vi "Start Preview.vi"(0 "Cluster In":T3, 1 "Start?":bool, 2 "Info":refnum<vi>, 3 "Stop":refnum<vi>, 4 "Pause":refnum<vi>, 5 "Run":refnum<vi>, 8 "Grab Window Image":refnum<vi>) -> (6 "Cluster Out":T3)   [LabVIEW 2010]
uses:
  System.Windows.Forms
  drivers/DirectShow SDK/v10/DirectShow SDK.llb/DirectShow - Capture Device.ctl
  D:/Projekte/Promotion/Scripts/LabView/drivers/DirectShow SDK/lib/DirectShowLib-2005.dll
  drivers/DirectShow SDK/lib/DirectShowLib-2005.dll
  drivers/DirectShow SDK/v10/DirectShow SDK.llb/DirectShow - Media State.ctl
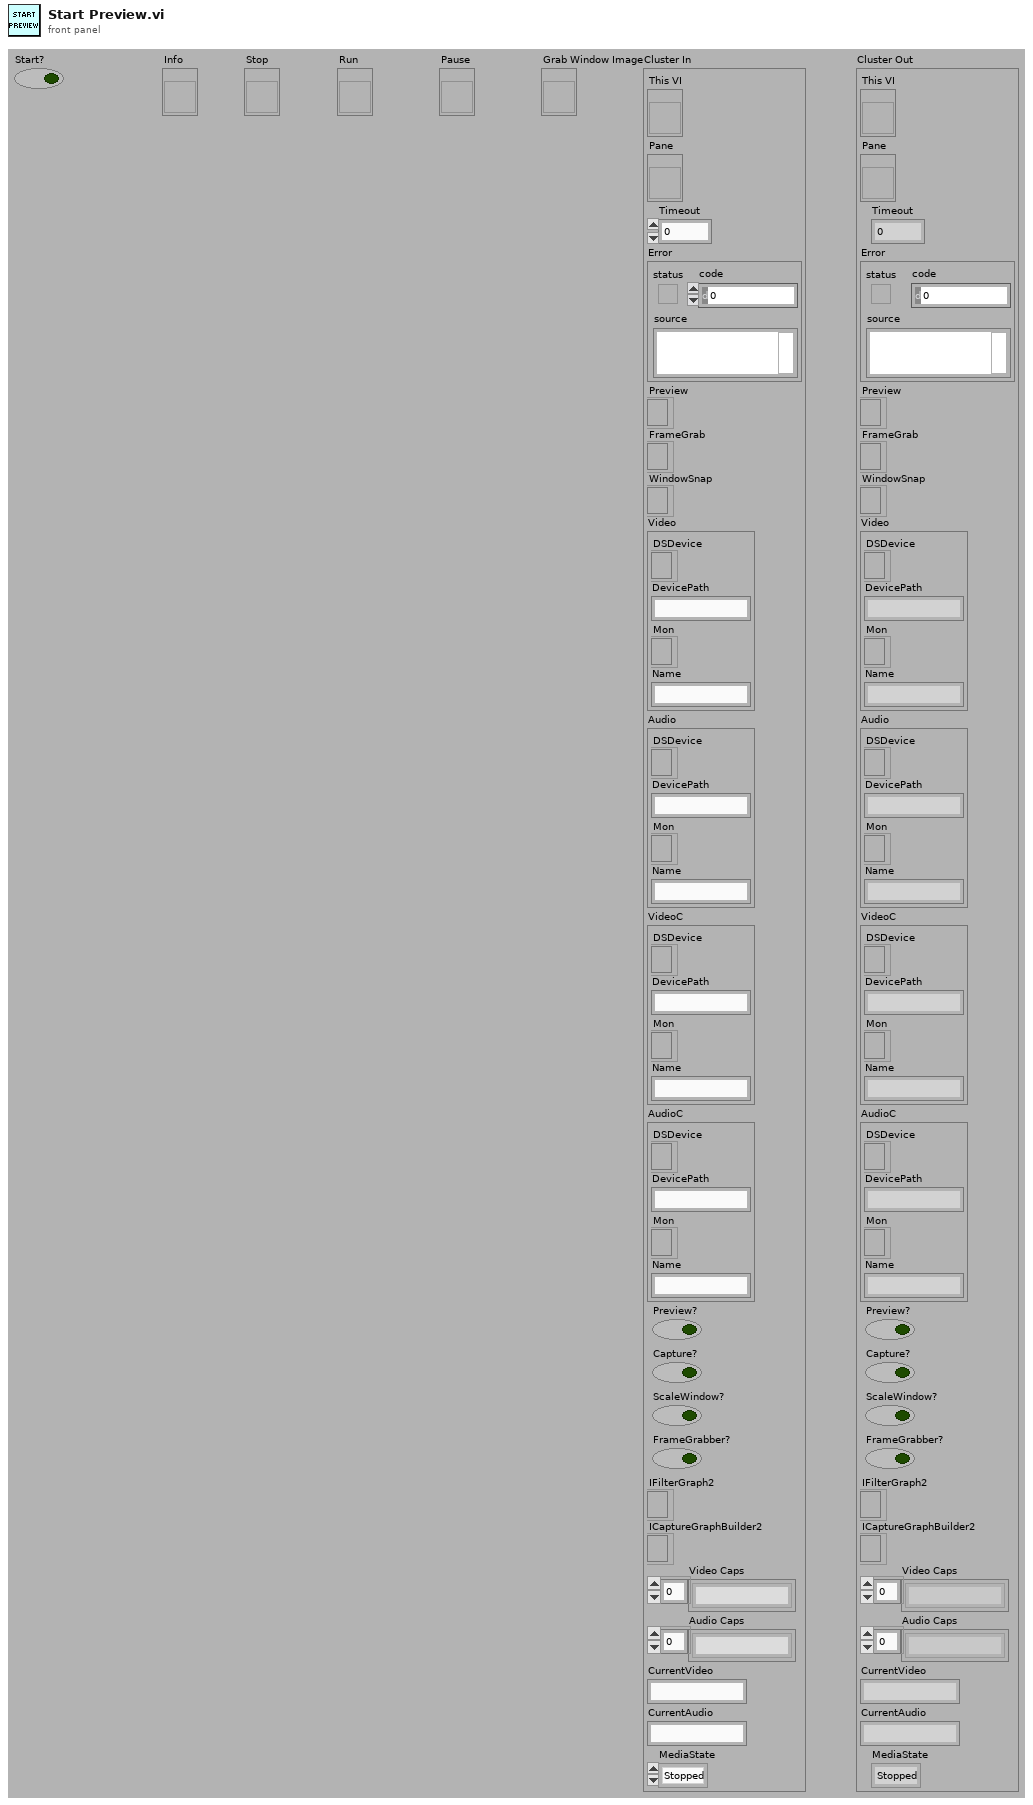
[diagram p1: front panel]
types:
  T1 = typedef "DirectShow - Capture Device.ctl" = cluster{"DSDevice":refnum<k24>, "DevicePath":string, "Mon":refnum<k24>, "Name":string}
  T2 = typedef "DirectShow - Media State.ctl" = enum16{"Stopped", "Playing", "Paused", "Recording"}
  T3 = cluster{"This VI":refnum<vi>, "Pane":refnum<vi>, "Timeout":i32, "Error":errorcluster, "Preview":refnum<k24>, "FrameGrab":refnum<k24>, "WindowSnap":refnum<k24>, "Video":T1, "Audio":T1, "VideoC":T1, "AudioC":T1, "Preview?":bool, "Capture?":bool, "ScaleWindow?":bool, "FrameGrabber?":bool, "IFilterGraph2":refnum<k24>, "ICaptureGraphBuilder2":refnum<k24>, "Video Caps":string[], "Audio Caps":string[], "CurrentVideo":string, "CurrentAudio":string, "MediaState":T2}
  T4 = enum8{"Enabled", "Disabled", "Disabled and Grayed Out"}
  T5 = typedef "LVRectTypeDef.ctl" = cluster{"left":i16, "top":i16, "right":i16, "bottom":i16}
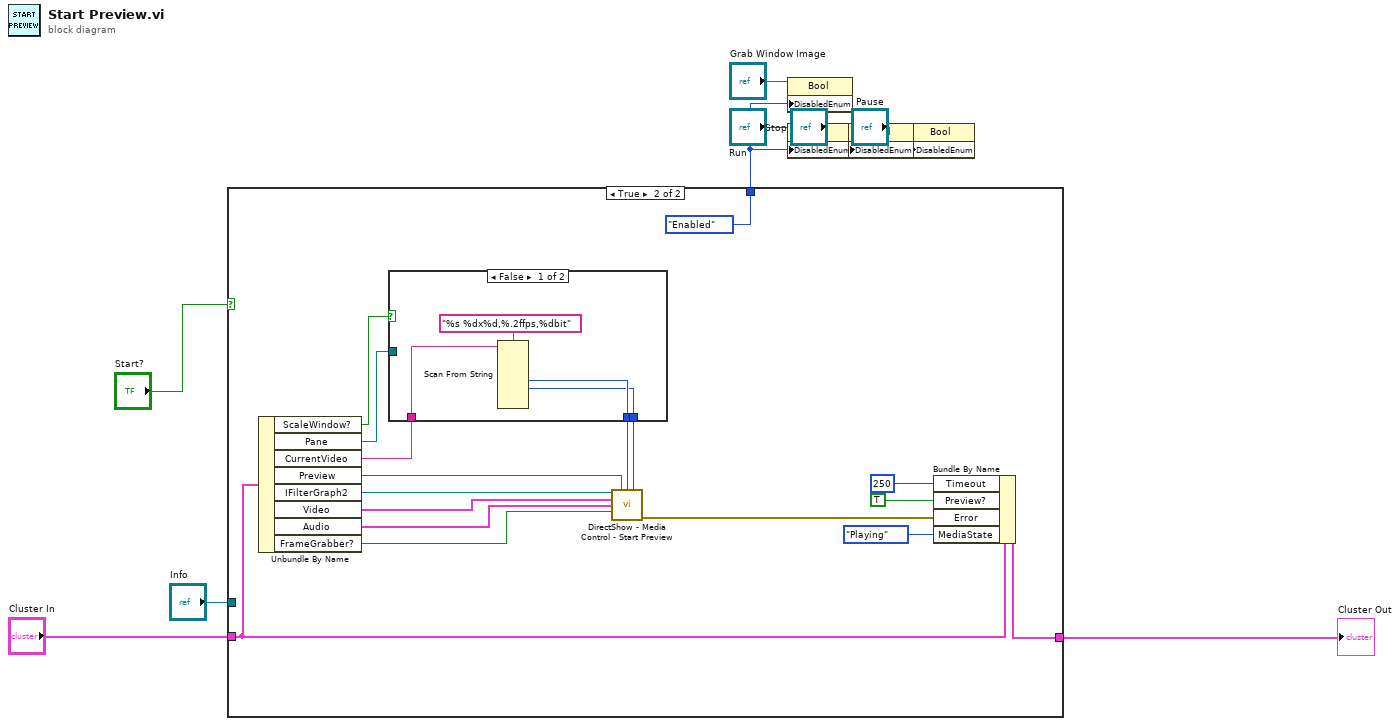
[diagram p0: block diagram]
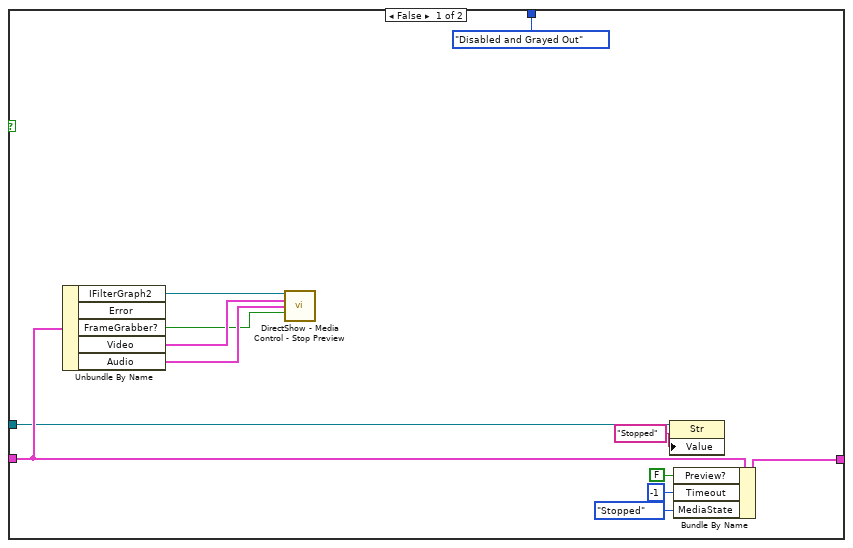
[diagram p2: hidden frame]
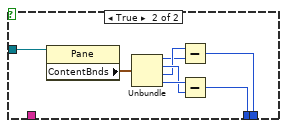
[diagram p3: hidden frame]
diagram:
  n1 = case shown="True" "Start?" {
    tunnel: [w21 w38] -> w7
    tunnel: [T4."Disabled and Grayed Out" ("Disabled") T4."Enabled" ("Disabled")] -> w6
    tunnel: "Cluster In" -> [w11 w22]
    tunnel: "Info" -> [w10 _]
    frame False {
      n2 = Unbundle By Name(w11) -> ("IFilterGraph2"=w16:refnum<k24>, "FrameGrabber?"=w13:bool, "Video"=w15:T1, "Audio"=w14:T1)  [unwired: 1 out]
      n3 = call "DirectShow - Media Control - Stop Preview.vi"("IFilterGraph2"=w16, "Video"=w15, "Audio"=w14, "FrameGrabber?"=w13) -> ()  [unwired: 10 in, 2 out]
      n4 = property class="Str"(reference=w10, "Value"="Stopped" ("Info")) -> ()  [unwired: 1 in, 2 out]
      n5 = Bundle By Name(cluster=w11, "Preview?"=FALSE, "Timeout"=-1, "MediaState"=DirectShow_-_Media_State."Stopped") -> (w21:T3)
    }
    frame True {
      n6 = Unbundle By Name(w22) -> ("ScaleWindow?"=w35:bool, "Pane"=w34:refnum<vi>, "CurrentVideo"=w33:string, "Preview"=w28:refnum<k24>, "IFilterGraph2"=w27:refnum<k24>, "Video"=w26:T1, "Audio"=w25:T1, "FrameGrabber?"=w24:bool)
      n7 = case shown="False" w35 {
        tunnel: w34 -> [_ w45]
        tunnel: [w40 w44] -> w30
        tunnel: [w39 w43] -> w29
        tunnel: w33 -> [w41 _]
        frame False {
          n8 = Scan From String(format string="%s %dx%d,%.2ffps,%dbit", input string=w41) -> (output 2=w40:i32, output 3=w39:i32)  [unwired: 10 in, 3 out]
        }
        frame True {
          n9 = property class="Pane"(reference=w45) -> ("ContentBnds"=w50:T5)  [unwired: 1 in, 2 out]
          n10 = Unbundle(w50) -> ("left"=w46:i16, "top"=w48:i16, "right"=w47:i16, "bottom"=w49:i16)
          n11 = Subtract(x=w47, y=w46) -> (x-y=w43:i16)
          n12 = Subtract(x=w49, y=w48) -> (x-y=w44:i16)
        }
      }
      n13 = call "DirectShow - Media Control - Start Preview.vi"("IFilterGraph2"=w27, "PictureBox"=w28, "width"=w30, "height"=w29, "Video"=w26, "Audio"=w25, "FrameGrabber?"=w24) -> ("error out"=w31:errorcluster)  [unwired: 7 in, 1 out]
      n14 = Bundle By Name(cluster=w22, "Timeout"=250, "Preview?"=TRUE, "Error"=w31, "MediaState"=DirectShow_-_Media_State."Playing") -> (w38:T3)
    }
  }
  "Cluster Out" <- w7
  n15 = property on="Property Node" class="Bool"(reference="Grab Window Image", "DisabledEnum"=w6) -> ()  [unwired: 1 in, 2 out]
  n16 = property on="Property Node" class="Bool"(reference="Run", "DisabledEnum"=w6) -> ()  [unwired: 1 in, 2 out]
  n17 = property on="Property Node" class="Bool"(reference="Stop", "DisabledEnum"=w6) -> ()  [unwired: 1 in, 2 out]
  n18 = property on="Property Node" class="Bool"(reference="Pause", "DisabledEnum"=w6) -> ()  [unwired: 1 in, 2 out]
